vi "test_libssh2_session_banner_set.vi"() -> ()   [LabVIEW 2017, in "integration_tests.lvlib"]
uses:
  integration_tests.lvlib
  libssh2/libssh2_session_handshake_tcp.vi
  libssh2/libssh2_init_default.vi
  libssh2/libssh2_session_init_ex.vi
  <vilib>/Utility/tcp.llb/TCP Get Raw Net Object.vi
  libssh2/libssh2_session_handshake_socket.vi
  libssh2/libssh2.lvlib
  support/support.lvlib
  <vilib>/PNR/Transparent Assertions/Transparent Assertions/Transparent Assertions.lvlib
panel:
  out "error out":errorcluster
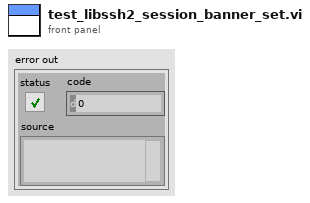
[diagram p1: front panel]
types:
  T1 = typedef "libssh2.lvlib/Session Refnum.ctl" = refnum<k1>
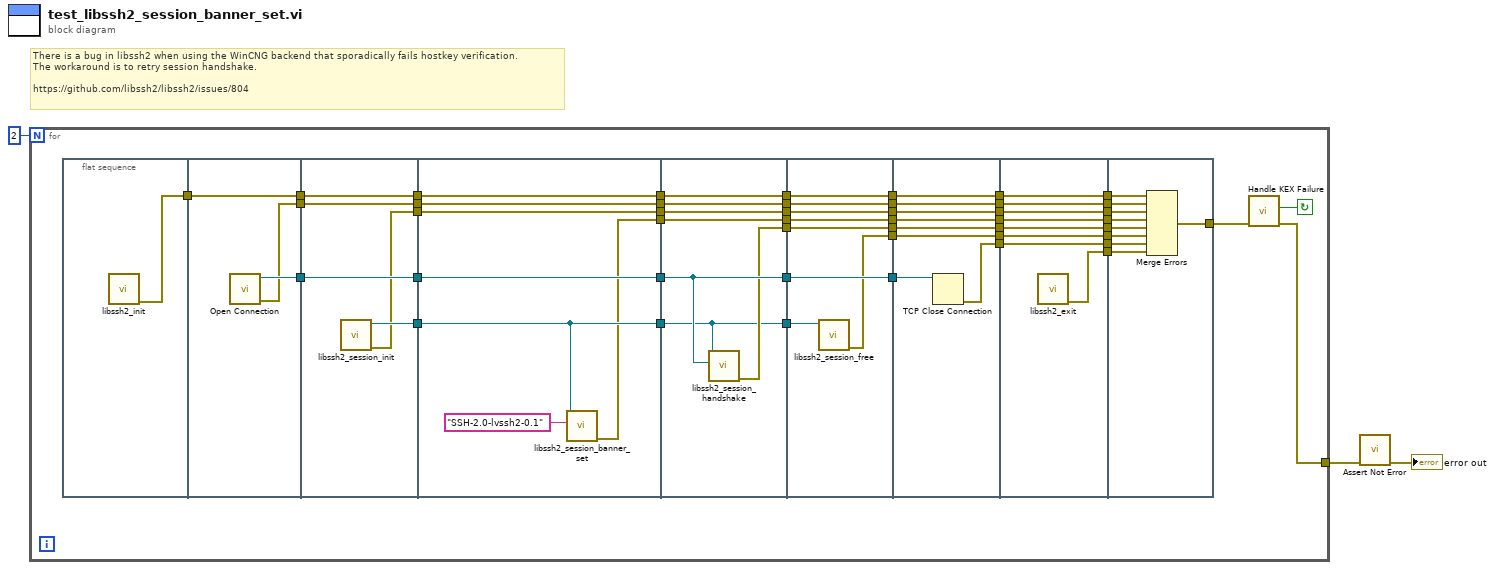
[diagram p0: block diagram]
diagram:
  # "There is a bug in libssh2 when using the WinCNG backend that sporadically fails hostkey verification.\nThe workaround is to retry session handshake.\n\nhttps://github.com/libssh2/libssh2/issues/804"
  n1 = for {
    N: 2 -> [_]
    tunnel: [w9] -> w2
    stop <- w10 continue-if-true
    n2 = flat-sequence {
      tunnel: [w51] -> w50
      tunnel: [w54] -> w49
      tunnel: w50 -> [w53]
      tunnel: [w53] -> w48
      tunnel: [w52] -> w47
      tunnel: w49 -> [w59]
      tunnel: [w59] -> w46
      tunnel: w48 -> [w58]
      tunnel: [w58] -> w45
      tunnel: w47 -> [w57]
      tunnel: [w57] -> w44
      tunnel: [w56] -> w43
      tunnel: [w55] -> w42
      tunnel: w46 -> [w66]
      tunnel: [w66] -> w41
      tunnel: w45 -> [w65]
      tunnel: [w65] -> w40
      tunnel: w44 -> [w64]
      tunnel: [w64] -> w39
      tunnel: w43 -> [w62]
      tunnel: [w62] -> w38
      tunnel: w42 -> [w63]
      tunnel: [w63] -> w37
      tunnel: [w60] -> w8
      tunnel: w41 -> [w70]
      tunnel: [w70] -> w36
      tunnel: w40 -> [w73]
      tunnel: [w73] -> w35
      tunnel: w39 -> [w72]
      tunnel: [w72] -> w34
      tunnel: w38 -> [w68]
      tunnel: w37 -> [w71]
      tunnel: [w71] -> w33
      tunnel: [w69] -> w32
      tunnel: [w68] -> w31
      tunnel: w8 -> [w67]
      tunnel: [w67] -> w7
      tunnel: w36 -> [w81]
      tunnel: [w81] -> w30
      tunnel: w35 -> [w80]
      tunnel: [w80] -> w29
      tunnel: w34 -> [w79]
      tunnel: [w79] -> w28
      tunnel: w33 -> [w78]
      tunnel: [w78] -> w27
      tunnel: w32 -> [w77]
      tunnel: [w77] -> w26
      tunnel: [w76] -> w25
      tunnel: w31 -> [w75]
      tunnel: w7 -> [w74]
      tunnel: [w74] -> w6
      tunnel: w30 -> [w89]
      tunnel: w29 -> [w88]
      tunnel: [w88] -> w24
      tunnel: w28 -> [w87]
      tunnel: [w87] -> w23
      tunnel: [w86] -> w22
      tunnel: w27 -> [w85]
      tunnel: [w85] -> w21
      tunnel: w26 -> [w84]
      tunnel: [w84] -> w20
      tunnel: [w83] -> w19
      tunnel: w25 -> [w83]
      tunnel: w6 -> [w82]
      tunnel: [w82] -> w5
      tunnel: w24 -> [w97]
      tunnel: [w97] -> w18
      tunnel: w23 -> [w96]
      tunnel: [w96] -> w17
      tunnel: w22 -> [w95]
      tunnel: [w95] -> w16
      tunnel: [w94] -> w15
      tunnel: w21 -> [w93]
      tunnel: [w93] -> w14
      tunnel: w20 -> [w92]
      tunnel: [w92] -> w13
      tunnel: [w91] -> w12
      tunnel: w19 -> [w91]
      tunnel: w5 -> [w90]
      tunnel: [w90] -> w4
      tunnel: w18 -> [w106]
      tunnel: w17 -> [w105]
      tunnel: w16 -> [w104]
      tunnel: w15 -> [w103]
      tunnel: w14 -> [w102]
      tunnel: w13 -> [w101]
      tunnel: w12 -> [w100]
      tunnel: [w99] -> w11
      tunnel: w4 -> [w98]
      frame #0 {
        n3 = call-poly "libssh2_init.vi"() -> ("error out"=w51:errorcluster)  [unwired: 11 in]
      }
      frame #1 {
        n4 = call "Open Connection.vi"() -> ("error out"=w52:errorcluster, "connection ID"=w54:refnum<k5>)  [unwired: 10 in]
      }
      frame #2 {
        n5 = call "libssh2_session_init.vi"() -> ("error out"=w55:errorcluster, "session"=w56:T1)  [unwired: 10 in]
      }
      frame #3 {
        n6 = call "libssh2_session_banner_set.vi"("banner"="SSH-2.0-lvssh2-0.1", "session"=w62) -> ("error out"=w60:errorcluster)  [unwired: 9 in]
      }
      frame #4 {
        n7 = call-poly "libssh2_session_handshake.vi"("tcp connection"=w70, "session"=w68) -> ("error out"=w69:errorcluster)  [unwired: 9 in]
      }
      frame #5 {
        n8 = call "libssh2_session_free.vi"("session"=w75) -> ("error out"=w76:errorcluster)  [unwired: 10 in]
      }
      frame #6 {
        n9 = TCP Close Connection(connection ID=w89) -> (error out=w86:errorcluster)  [unwired: 2 in, 1 out]
      }
      frame #7 {
        n10 = call "libssh2_exit.vi"() -> ("error out"=w94:errorcluster)  [unwired: 11 in]
      }
      frame #8 {
        n11 = Merge Errors(w106, w105, w102, w98, w101, w100, w104, w103) -> (w99:errorcluster)
      }
    }
    n12 = call "Handle KEX Failure.vi"("error in (no error)"=w11) -> ("error out"=w9:errorcluster, "KEX Failure"=w10:bool)  [unwired: 9 in]
  }
  n13 = call <vilib>:"Assert Not Error.vi"("error in (no error)"=w2) -> ("error out"=→"error out":errorcluster)  [unwired: 10 in]
